vi "Default Data.vi"(2 "Num Rows":i32, 3 "Device in":refnum<class "Device.lvclass">) -> (0 "Default Data":string[][](table), 1 "Device out":refnum<class "Device.lvclass">)   [LabVIEW 2013, in "Device.lvclass"]
doc: "Fill existing rows with 0's, unless specifically overridden."
uses:
  Device.lvclass
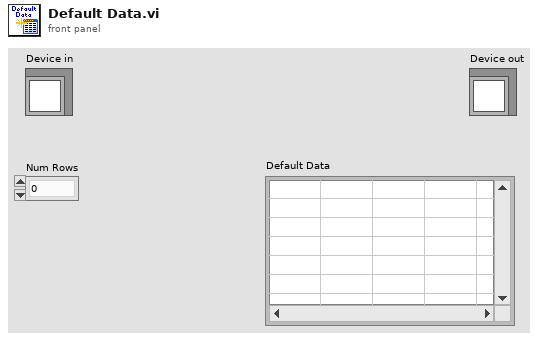
[diagram p1: front panel]
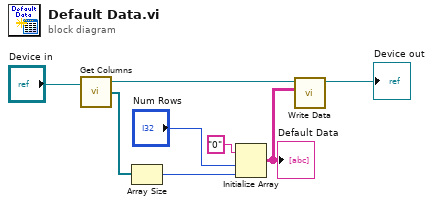
[diagram p0: block diagram]
diagram:
  n1 = call-dynamic "Get Columns.vi"("Device in"="Device in") -> ("Device out"=w7:refnum<class "Device.lvclass">, "Columns"=w4:refnum<class "Column.lvclass">[])  [unwired: 1 in, 1 out]
  n2 = Array Size(array=w4) -> (size(s)=w3:i32)
  n3 = Initialize Array("0", "Num Rows", w3) -> (w2:string[][])
  "Default Data" <- w2
  n4 = call-dynamic "Write Data.vi"("Data"=w2, "Device in"=w7) -> ("Device Out"=→"Device out":refnum<class "Device.lvclass">)  [unwired: 8 in, 1 out]
